vi "Reserve SPI.vi"(7 "SPI Pins":T1={"TX GPIO"=-1, "RX GPIO"=-1, "SCK GPIO"=6}, 8 "error in (no error)":errorcluster, 9 "Purpose":string, 10 "SPI #":T3=-1, 11 "Session in":refnum<class "Session.lvclass">) -> (0 "error out":errorcluster, 3 "Session out":refnum<class "Session.lvclass">)   [LabVIEW 2024, in "CTI.lvlib" / "Session.lvclass"]
uses:
  Session.lvclass
  SPI Number.ctl
  SPI Pins.ctl
  GPIO Number.ctl
  Resource/Resource.lvclass/Resource.ctl
  Session.lvclass/Session.ctl
  dcef0d26-6755-4235-b060-6b0e00c3d74f.vi
  dcef0d26-6755-4235-b060-6b0e00c3d74f.vi/685f7f19-b444-4620-8f66-e6e2ddd64bb8.vi
  SPI/SPI.lvclass
  C:/Users/nkirchne/Documents/~SANDBOX/Electronics Workflow/build/ForPort/CTI/Resource/Resource.lvclass
  Generate Error.vi
  Resource/Resource.lvclass
  CTI.lvlib
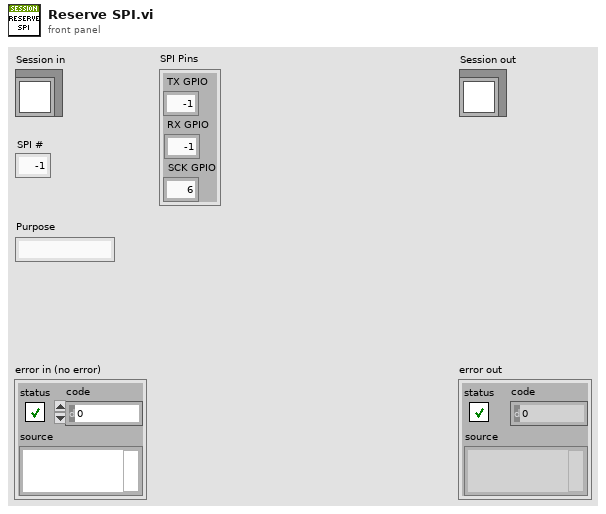
[diagram p1: front panel]
types:
  T1 = typedef "CTI.lvlib/SPI Pins.ctl" = cluster{"TX GPIO":T2, "RX GPIO":T2, "SCK GPIO":T2}
  T2 = typedef "CTI.lvlib/GPIO Number.ctl" = i8
  T3 = typedef "CTI.lvlib/SPI Number.ctl" = i8
  T4 = typedef "CTI.lvlib/Session.lvclass/Resources.ctl" = cluster{"GPIO":map{T2, refnum<class "GPIO.lvclass">}, "AI":map{T5, refnum<class "AI.lvclass">}, "PWM":map{T2, refnum<class "PWM.lvclass">}, "UART":map{T6, refnum<class "UART.lvclass">}, "I2C":map{T7, refnum<class "I2C.lvclass">}, "SPI":map{T3, refnum<class "SPI.lvclass">}, "SPI CS":map{T2, refnum<class "SPI CS.lvclass">}}
  T5 = typedef "CTI.lvlib/ADC Number.ctl" = i8
  T6 = typedef "CTI.lvlib/UART Number.ctl" = i8
  T7 = typedef "CTI.lvlib/I2C Number.ctl" = i8
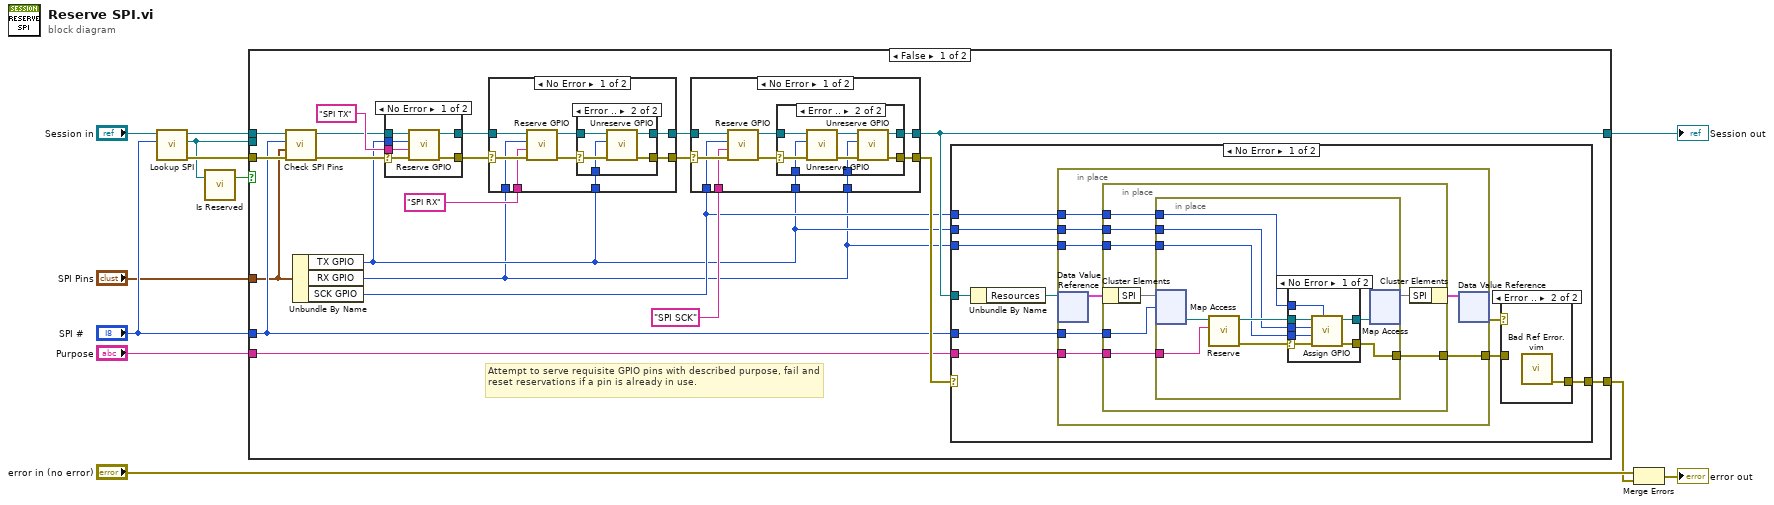
[diagram p0: block diagram]
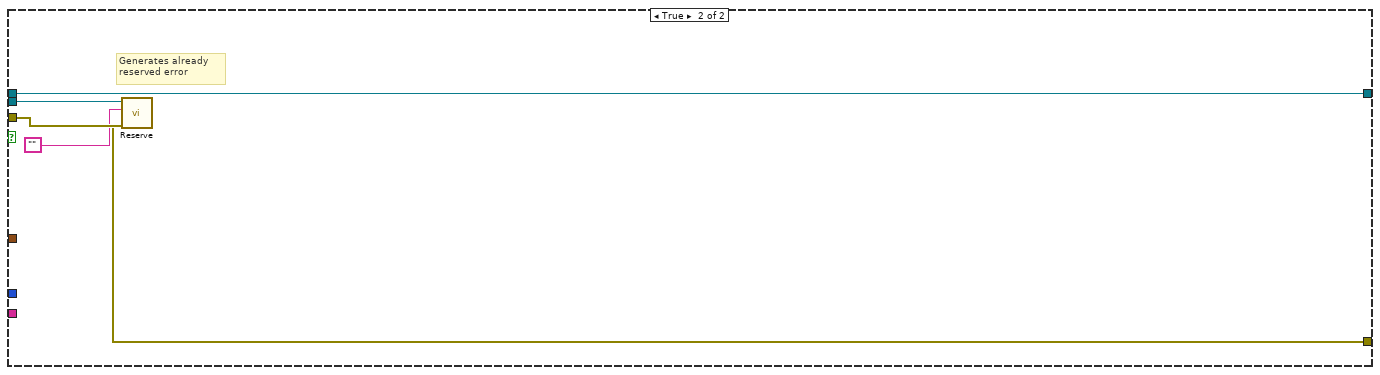
[diagram p10: hidden frame]
diagram:
  n1 = call "Lookup SPI.vi"("SPI #"="SPI #", "Session in"="Session in") -> ("error out"=w12:errorcluster, "SPI"=w1:refnum<class "SPI.lvclass">, "Session out"=w6:refnum<class "Session.lvclass">)  [unwired: 7 in]
  n2 = call "Is Reserved.vi"("Resource in"=w1) -> ("Reserved"=w2:bool)  [unwired: 6 in]
  n3 = case shown="False" w2 {
    tunnel: w12 -> [w30 w131]
    tunnel: "Purpose" -> [w29 _]
    tunnel: [w28 w129] -> w7
    tunnel: w6 -> [w19 w130]
    tunnel: "SPI #" -> [w17 _]
    tunnel: "SPI Pins" -> [w16 _]
    tunnel: [w22 w130] -> w3
    tunnel: w1 -> [_ w132]
    frame False {
      # "Attempt to serve requisite GPIO pins with described purpose, fail and reset reservations if a pin is already in use."
      n4 = call "Check SPI Pins.vi"("error in (no error)"=w30, "SPI Pins"=w16, "SPI #"=w17, "Session in"=w19) -> ("error out"=w20:errorcluster, "Session out"=w18:refnum<class "Session.lvclass">)  [unwired: 6 in]
      n5 = Unbundle By Name(w16) -> ("TX GPIO"=w14:T2, "RX GPIO"=w13:T2, "SCK GPIO"=w15:T2)
      n6 = case shown="No Error" w20 {
        selector: w20 -> [w34 w39]
        tunnel: [w38 w39] -> w31
        tunnel: "SPI TX" ("Purpose") -> [w37 _]
        tunnel: [w36 w40] -> w26
        tunnel: w14 -> [w35 _]
        tunnel: w18 -> [w33 w40]
        frame No Error {
          n7 = call "Reserve GPIO.vi"("error in (no error)"=w34, "Purpose"=w37, "GPIO #"=w35, "Session in"=w33) -> ("error out"=w38:errorcluster, "Session out"=w36:refnum<class "Session.lvclass">)  [unwired: 6 in]
        }
        frame Error {
        }
      }
      n8 = case shown="No Error" w31 {
        selector: w31 -> [w49 w57]
        tunnel: [w42 w57] -> w23
        tunnel: w26 -> [w48 w58]
        tunnel: [w43 w58] -> w24
        tunnel: w13 -> [w47 _]
        tunnel: "SPI RX" ("Purpose") -> [w46 _]
        tunnel: w14 -> [w41 _]
        frame No Error {
          n9 = call "Reserve GPIO.vi"("error in (no error)"=w49, "Purpose"=w46, "GPIO #"=w47, "Session in"=w48) -> ("error out"=w45:errorcluster, "Session out"=w44:refnum<class "Session.lvclass">)  [unwired: 6 in]
          n10 = case shown="Error .." w45 {
            selector: w45 -> [w50 w55]
            tunnel: w44 -> [w51 w56]
            tunnel: [w51 w52] -> w43
            tunnel: [w50 w53] -> w42
            tunnel: w41 -> [_ w54]
            frame No Error {
            }
            frame Error {
              n11 = call "Unreserve GPIO.vi"("error in (no error)"=w55, "GPIO #"=w54, "Session in"=w56) -> ("error out"=w53:errorcluster, "Session out"=w52:refnum<class "Session.lvclass">)  [unwired: 7 in]
            }
          }
        }
        frame Error {
        }
      }
      n12 = case shown="No Error" w23 {
        selector: w23 -> [w68 w79]
        tunnel: [w61 w79] -> w32
        tunnel: w24 -> [w67 w80]
        tunnel: [w62 w80] -> w22
        tunnel: w15 -> [w66 _]
        tunnel: "SPI SCK" ("Purpose") -> [w65 _]
        tunnel: w14 -> [w60 _]
        tunnel: w13 -> [w59 _]
        frame No Error {
          n13 = call "Reserve GPIO.vi"("error in (no error)"=w68, "Purpose"=w65, "GPIO #"=w66, "Session in"=w67) -> ("error out"=w64:errorcluster, "Session out"=w63:refnum<class "Session.lvclass">)  [unwired: 6 in]
          n14 = case shown="Error .." w64 {
            selector: w64 -> [w69 w77]
            tunnel: w63 -> [w70 w78]
            tunnel: [w70 w72] -> w62
            tunnel: [w69 w73] -> w61
            tunnel: w60 -> [_ w76]
            tunnel: w59 -> [_ w71]
            frame No Error {
            }
            frame Error {
              n15 = call "Unreserve GPIO.vi"("error in (no error)"=w77, "GPIO #"=w76, "Session in"=w78) -> ("error out"=w74:errorcluster, "Session out"=w75:refnum<class "Session.lvclass">)  [unwired: 7 in]
              n16 = call "Unreserve GPIO.vi"("error in (no error)"=w74, "GPIO #"=w71, "Session in"=w75) -> ("error out"=w73:errorcluster, "Session out"=w72:refnum<class "Session.lvclass">)  [unwired: 7 in]
            }
          }
        }
        frame Error {
        }
      }
      n17 = case shown="No Error" w32 {
        selector: w32 -> [_ w127]
        tunnel: w29 -> [w89 _]
        tunnel: [w86 w127] -> w28
        tunnel: w17 -> [w85 _]
        tunnel: w22 -> [w84 _]
        tunnel: w15 -> [w83 _]
        tunnel: w14 -> [w82 _]
        tunnel: w13 -> [w81 _]
        frame No Error {
          n18 = Unbundle By Name(w84) -> ("Resources"=w90:refnum<data-value>)
          n19 = in-place {
            in-place-border: w85 -> [w98]
            in-place-border: w89 -> [w97]
            in-place-border: [w96] -> w88
            in-place-border: w83 -> [w93]
            in-place-border: w82 -> [w92]
            in-place-border: w81 -> [w91]
            n20 = in-place-dvr #1(w90) -> (w94:T4)  [unwired: 1 out]
            n21 = in-place {
              in-place-border: w98 -> [w105]
              in-place-border: w97 -> [w104]
              in-place-border: [w103] -> w96
              in-place-border: w93 -> [w101]
              in-place-border: w92 -> [w100]
              in-place-border: w91 -> [w99]
              n22 = in-place-cluster #2(w94) -> ("SPI"=w106:map{T3, refnum<class "SPI.lvclass">})
              n23 = in-place {
                in-place-border: w104 -> [w114]
                in-place-border: [w107] -> w103
                in-place-border: w101 -> [w111]
                in-place-border: w100 -> [w110]
                in-place-border: w99 -> [w109]
                n24 = in-place-map #3(w106, w105) -> (w115:refnum<class "SPI.lvclass">)  [unwired: 1 in, 1 out]
                n25 = call "Reserve.vi"("Purpose"=w114, "Resource in"=w115) -> ("error out"=w108:errorcluster, "Resource out"=w113:refnum<class "SPI.lvclass">)  [unwired: 8 in]
                n26 = case shown="No Error" w108 {
                  selector: w108 -> [w119 w123]
                  tunnel: w113 -> [w122 w124]
                  tunnel: [w121 w124] -> w112
                  tunnel: w111 -> [w120 _]
                  tunnel: w110 -> [w117 _]
                  tunnel: w109 -> [w116 _]
                  tunnel: [w118 w123] -> w107
                  frame No Error {
                    n27 = call "Assign GPIO.vi"("SCK"=w120, "error in (no error)"=w119, "RX"=w116, "TX"=w117, "SPI in"=w122) -> ("error out"=w118:errorcluster, "SPI out"=w121:refnum<class "SPI.lvclass">)  [unwired: 5 in]
                  }
                  frame Error {
                  }
                }
                n28 = in-place-map #3(w112) -> (w102:map{T3, refnum<class "SPI.lvclass">})  [unwired: 1 in, 2 out]
              }
              n29 = in-place-cluster #2("SPI"=w102) -> (w95:T4)
            }
            n30 = in-place-dvr #1(w95) -> (w87:errorcluster)  [unwired: 1 out]
          }
          n31 = case shown="Error .." w87 {
            tunnel: w88 -> [w125 _]
            tunnel: [w125 w126] -> w86
            frame No Error {
            }
            frame Error {
              n32 = call "Bad Ref Error.vim"() -> ("error out"=w126:errorcluster)  [unwired: 10 in, 1 out]
            }
          }
        }
        frame Error {
          # "Error generated reserving GPIO Pin(s) or looking up I2C #"
        }
      }
    }
    frame True {
      # "Generates already reserved error"
      n33 = call "Reserve.vi"("error in (no error)"=w131, "Purpose"="", "Resource in"=w132) -> ("error out"=w129:errorcluster)  [unwired: 7 in, 1 out]
    }
  }
  "Session out" <- w3
  n34 = Merge Errors("error in (no error)", w7) -> (→"error out":errorcluster)
